vi "DO Write.vi"(8 "error in (no error)":errorcluster, 10 "Digital Output":bool, 11 "Valve in":refnum<class "Valve.lvclass">) -> (0 "error out":errorcluster)   [LabVIEW 2021, in "Valve.lvlib" / "Valve.lvclass"]
uses:
  Valve.lvclass
  Valve.lvclass/Valve.ctl
  DAQ-arch/Digital Output On Demand/Digital Output On Demand/Digital Output On Demand.lvclass
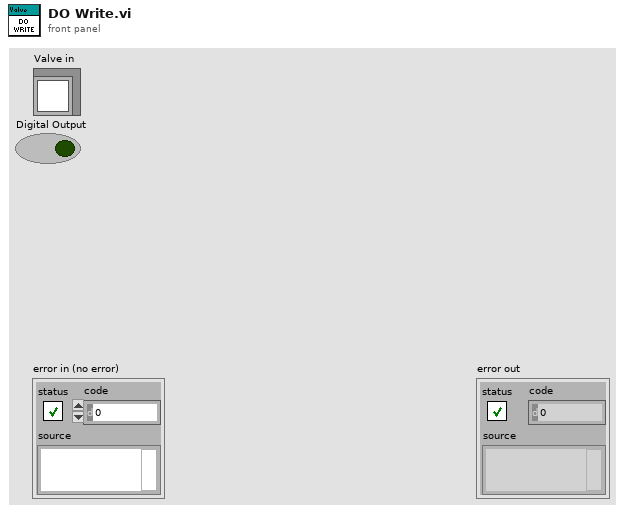
[diagram p1: front panel]
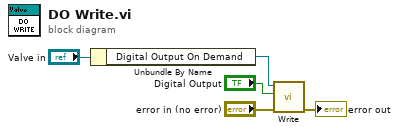
[diagram p0: block diagram]
diagram:
  n1 = Unbundle By Name("Valve in") -> ("Digital Output On Demand"=w4:refnum<class "Digital Output On Demand.lvclass">)
  n2 = call "Write.vi"("error in (no error)"="error in (no error)", "Digital Output"="Digital Output", "Digital Output On Demand in"=w4) -> ("error out"=→"error out":errorcluster)  [unwired: 8 in]
